vi "OxITC503 _Config_ Gas Flow.vi"(2 "error in":errorcluster, 3 "Gas Flow Value":dbl format="%.2f", 4 "VISA session":refnum<visa-resource-name>) -> (0 "error out (no error)":errorcluster, 1 "VISA session":refnum<visa-resource-name>)   [LabVIEW 2013]
doc: "Sets the GAS FLOW to a defined value nnn (for use with AutoGFS)."
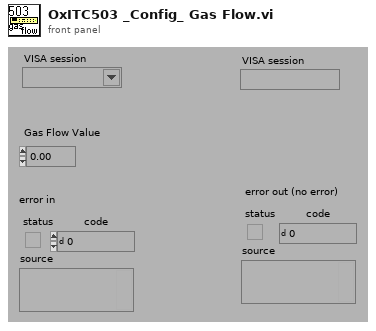
[diagram p1: front panel]
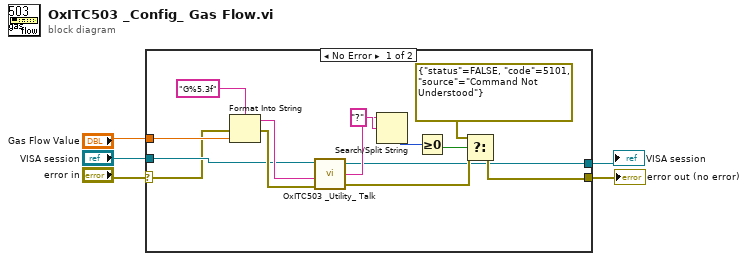
[diagram p0: block diagram]
diagram:
  n1 = case shown="No Error" "error in" {
    selector: "error in" -> [w6 w20]
    tunnel: [w18 w20] -> w5
    tunnel: "Gas Flow Value" -> [w10 _]
    tunnel: [w8 w21] -> w3
    tunnel: "VISA session" -> [w7 w21]
    frame No Error {
      n2 = Format Into String(format string="G%5.3f" ("Format String"), error in=w6, w10) -> (resulting string=w11:string, error out=w12:errorcluster)  [unwired: 1 in]
      n3 = call "OxITC503 _Utility_ Talk.vi"("VISA session"=w7, "Command"=w11, "error in (no error)"=w12) -> ("VISA session"=w8:refnum<visa-resource-name>, "read buffer"=w13:string, "error out (no error)"=w17:errorcluster)  [unwired: 2 in]
      n4 = Search/Split String(string=w13, search string/char (-)="?" ("search char (-)")) -> (offset of match=w15:i32)  [unwired: 1 in, 2 out]
      n5 = Greater Or Equal To 0?(x=w15) -> (x >= 0?=w16:bool)
      n6 = Select(t=errorcluster {"status"=FALSE, "code"=5101, "source"="Command Not Understood"}, s=w16, f=w17) -> (s? t:f=w18:errorcluster)
    }
    frame Error {
    }
  }
  "error out (no error)" <- w5
  "VISA session" <- w3
